vi "Read myTemp.vi"(6 "Reset Time":bool, 8 "error in (no error)":errorcluster, 9 "myTemp Setup":T1={"Offset Temp"=0.0, "Set Offset"=FALSE, "Calibration Data"=[{"Ka"=0.000739984, "Kb"=0.000278736, "Kc"=9.26322e-08}, {"Ka"=0.00073998, "Kb"=0.00027874, "Kc"=9.2632e-08}, {"Ka"=0.00073998, "Kb"=0.00027874, "Kc"=9.2632e-08}, {"Ka"=0.00073998, "Kb"=0.00027874, "Kc"=9.2632e-08}, {"Ka"=0.00073998, "Kb"=0.00027874, "Kc"=9.2632e-08}, {"Ka"=0.00073998, "Kb"=0.00027874, "Kc"=9.2632e-08}, {"Ka"=0.00073998, "Kb"=0.00027874, "Kc"=9.2632e-08}], "Chan Select"=[TRUE, TRUE, TRUE, FALSE, FALSE, FALSE, FALSE], "Clear Offsets"=FALSE, "Input Mode"=FALSE, "Chart History Length"=2000, "Use One K Set"=TRUE} {"Chart History Length" min=1 max=10000 step=1; "Calibration Data"."Kc" format="%#.4e"; "Calibration Data"."Kb" format="%#.4e"; "Calibration Data"."Ka" format="%#.4e"; "Offset Temp" min=-40.0 max=250.0 step=1.0}, 11 "task array in":refnum<k21>[](array[refnum])) -> (0 "error out":errorcluster, 1 "Elapsed Time":dbl, 2 "temperature values (°C)":dbl[](array[numeric]), 3 "task array out":refnum<k21>[](array[refnum]), 5 "XY Graph":cluster{"X":dbl[], "Y":dbl[]}[](array[cluster]))   [LabVIEW 2013]
doc: "This subVI is designed to control the multiplexor on the PITSCO myTemp so it can read in up to 7 temperature values. It use Steinhart non-linear scaling to convert the voltage measurements to temperature in °C."
uses:
  <vilib>/DAQmx/write.llb/DAQmx Write (Digital 1D Bool NChan 1Samp 1Line).vi
  <vilib>/DAQmx/read.llb/DAQmx Read (Analog 1D Wfm NChan NSamp).vi
  <vilib>/Analysis/baseanly.llb/Mean (DBL).vi
  <vilib>/DAQmx/miscellaneous.llb/DAQmx Fill In Error Info.vi
  <vilib>/Analysis/NI_AALBase.lvlib
panel:
  # "Select Temperature Channels to Display"
  # "Temp1"
  # "Temp2"
  # "Temp3"
  # "Temp4"
  # "Temp5"
  # "Temp6"
  # "Temp7"
  # "Null Temperature Setting"
  # "Calibration Coefficients"
  # "Temp1"
  # "Temp2"
  # "Temp3"
  # "Temp4"
  # "Temp5"
  # "Temp6"
  # "Temp7"
  # "Ka"
  # "Kb"
  # "Kc"
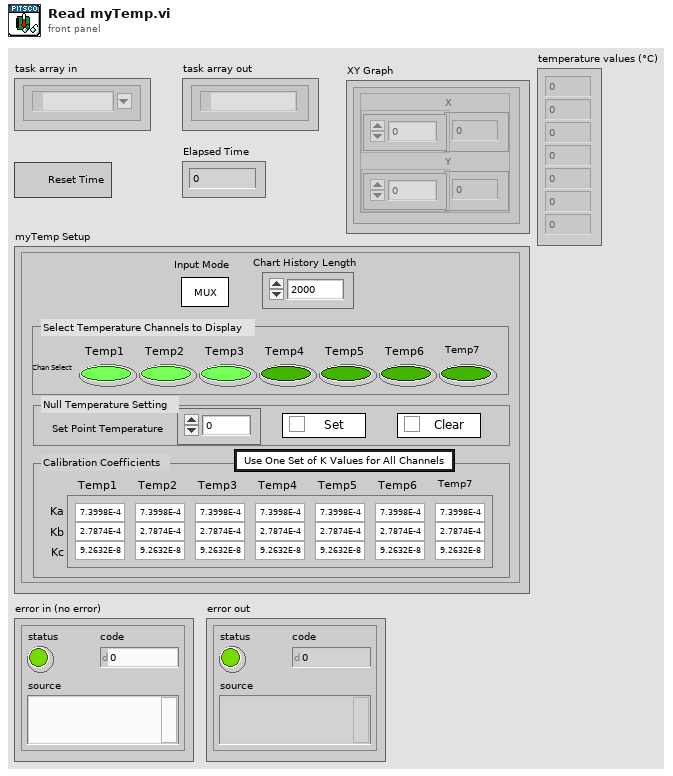
[diagram p1: front panel]
types:
  T1 = cluster{"Offset Temp":dbl, "Set Offset":bool, "Calibration Data":cluster{"Ka":dbl, "Kb":dbl, "Kc":dbl}[], "Chan Select":bool[], "Clear Offsets":bool, "Input Mode":bool, "Chart History Length":i32, "Use One K Set":bool}
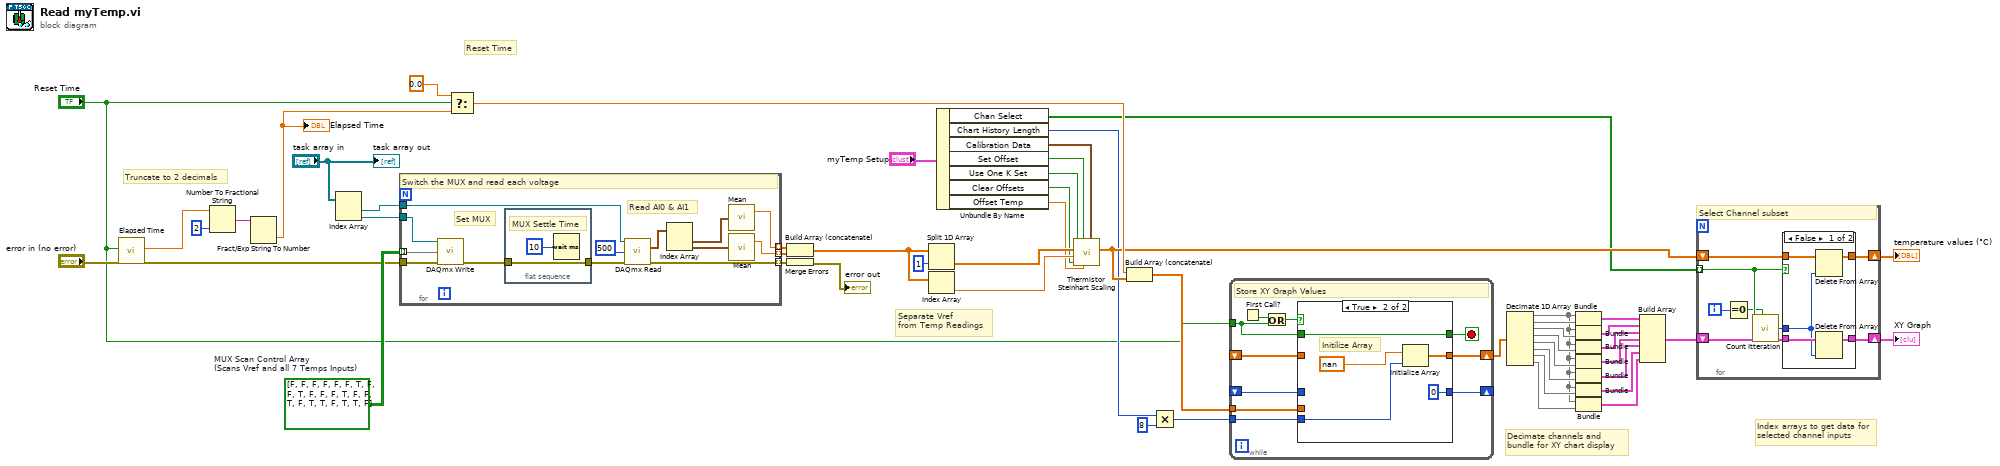
[diagram p0: block diagram]
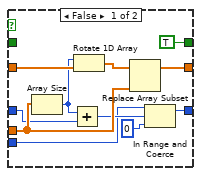
[diagram p2: hidden frame]
diagram:
  w37 = bool[][] [[FALSE, FALSE, FALSE, FALSE, FALSE, FALSE], [TRUE, FALSE, FALSE, TRUE, FALSE, FALSE], [FALSE, TRUE, FALSE, FALSE, TRUE, FALSE], [TRUE, TRUE, FALSE, TRUE, TRUE, FALSE]]  # MUX Scan Control Array (Scans Vref and all 7 Temps Inputs)
  # "Reset Time"
  # "Truncate to 2 decimals"
  # "Separate Vref\nfrom Temp Readings"
  # "Index arrays to get data for\nselected channel inputs"
  # "Decimate channels and \nbundle for XY chart display"
  n1 = call "Elapsed Time"("Reset"="Reset Time", "error in (no error)"="error in (no error)") -> ("Elapsed Time (s)"=w14:dbl, "error out"=w15:errorcluster)  [unwired: 10 in, 6 out]
  n2 = Number To Fractional String(number=w14, precision (6)=i16 2 ("precision (3)")) -> (F-format string=w17:string)  [unwired: 2 in]
  n3 = Fract/Exp String To Number(string=w17) -> (number=w8:dbl)  [unwired: 3 in, 1 out]
  "Elapsed Time" <- w8
  n4 = Index Array(array="task array in") -> (element #1=w6:refnum<k21>, element #2=w7:refnum<k21>)  [unwired: 2 in]
  n5 = for {
    tunnel: [w59] -> w39 mode=indexing
    tunnel: w37 -> [w58] mode=indexing
    tunnel: [w54] -> w41 mode=indexing
    tunnel: [w53] -> w40 mode=indexing
    tunnel: w15 -> [w61]
    tunnel: w7 -> [w65]
    tunnel: w6 -> [w63]
    # "Read AI0 & AI1"
    # "Set MUX"
    # "Switch the MUX and read each voltage"
    n6 = call-poly <vilib>:"DAQmx Write.vi"("task/channels in"=w65, "data"=w58, "error in"=w61) -> ("error out"=w60:errorcluster)  [unwired: 10 in, 2 out]
    n7 = flat-sequence {
      tunnel: w60 -> [w67]
      tunnel: [w67] -> w62
      frame #0 {
        # "MUX Settle Time"
        n8 = Wait (ms)(milliseconds to wait=u32 10) -> ()  [unwired: 1 out]
      }
    }
    n9 = call-poly <vilib>:"DAQmx Read.vi"("task/channels in"=w63, "number of samples per channel"=500, "error in"=w62) -> ("data"=w57:waveform(dbl)[], "error out"=w59:errorcluster)  [unwired: 10 in, 1 out]
    n10 = Index Array(array=w57) -> (element #1=w56:waveform(dbl), element #2=w55:waveform(dbl))  [unwired: 2 in]
    n11 = call-poly <vilib>:"Mean.vi"("X"=w56) -> ("mean"=w54:dbl)  [unwired: 1 out]
    n12 = call-poly <vilib>:"Mean.vi"("X"=w55) -> ("mean"=w53:dbl)  [unwired: 1 out]
  }
  n13 = Select(t=0.0, s="Reset Time", f=w8) -> (s? t:f=w51:dbl)
  n14 = Build Array (concatenate)(w41, w40) -> (w44:dbl[])
  n15 = Merge Errors(w39) -> (→"error out":errorcluster)
  n16 = Split 1D Array(array=w44, index=1) -> (second subarray=w42:dbl[])  [unwired: 1 out]
  n17 = Index Array(array=w44) -> (element=w46:dbl)  [unwired: 1 in]
  n18 = Unbundle By Name("myTemp Setup") -> ("Chan Select"=w20:bool[], "Chart History Length"=w21:i32, "Calibration Data"=w47:cluster{"Ka":dbl, "Kb":dbl, "Kc":dbl}[], "Set Offset"=w48:bool, "Use One K Set"=w43:bool, "Clear Offsets"=w18:bool, "Offset Temp"=w19:dbl)
  n19 = call "Thermistor Steinhart Scaling.vi"("Calibration Coefficients"=w47, "Set Point Temp"=w19, "Set"=w48, "Clear"=w18, "Vref"=w46, "Vt Measured"=w42, "Use One K Set"=w43) -> ("Temps"=w38:dbl[])  [unwired: 3 in, 1 out]
  n20 = Build Array (concatenate)(w51, w38) -> (w4:dbl[])
  n21 = Multiply(x=w21, y=8) -> (x*y=w2:i32)
  n22 = while {
    tunnel: w2 -> [w77]
    shift-right: [w76] -> w1
    shift-left: _ -> [w75]
    tunnel: w4 -> [w74]
    shift-right: [w70] -> _
    shift-left: _ -> [w69]
    tunnel: "Reset Time" -> [w68]
    stop <- w71 stop-if-true
    # "Store XY Graph Values"
    n23 = First Call?() -> (First Call?: T/F=w73:bool)
    n24 = Or(x=w73, y=w68) -> (x .or. y?=w72:bool)
    n25 = case shown="True" w72 {
      tunnel: w77 -> [w80 w93]
      tunnel: [w86 w91] -> w76
      tunnel: w75 -> [w88 _]
      tunnel: w74 -> [w85 _]
      tunnel: [TRUE w90] -> w71
      tunnel: w68 -> [_ w90]
      tunnel: [w78 0] -> w70
      tunnel: w69 -> [w83 _]
      frame False {
        n26 = Array Size(array=w85) -> (size(s)=w82:i32)
        n27 = Add(x=w82, y=w83) -> (x+y=w81:i32)
        n28 = Rotate 1D Array(1:w88, 2:w82) -> (0:w87:dbl[])
        n29 = Replace Array Subset(array=w87, new element=w85) -> (w86:dbl[])  [unwired: 1 in]
        n30 = In Range and Coerce(upper limit=w80, x=w81, lower limit=0) -> (coerced(x)=w78:i32)  [unwired: 1 out]
      }
      frame True {
        # "Initilize Array"
        n31 = Initialize Array(nan ("element"), w93) -> (w91:dbl[])
      }
    }
  }
  n32 = Decimate 1D Array(w1) -> (w22:dbl[], w23:dbl[], w24:dbl[], w25:dbl[], w26:dbl[], w27:dbl[], w28:dbl[], w29:dbl[])
  n33 = Bundle(w22, w23) -> (w30:cluster{dbl[], dbl[]})  [unwired: 1 in]
  n34 = Bundle(w22, w24) -> (w31:cluster{dbl[], dbl[]})  [unwired: 1 in]
  n35 = Bundle(w22, w25) -> (w32:cluster{dbl[], dbl[]})  [unwired: 1 in]
  n36 = Bundle(w22, w26) -> (w33:cluster{dbl[], dbl[]})  [unwired: 1 in]
  n37 = Bundle(w22, w27) -> (w34:cluster{dbl[], dbl[]})  [unwired: 1 in]
  n38 = Bundle(w22, w28) -> (w35:cluster{dbl[], dbl[]})  [unwired: 1 in]
  n39 = Bundle(w22, w29) -> (w36:cluster{dbl[], dbl[]})  [unwired: 1 in]
  n40 = Build Array(w30, w31, w32, w33, w34, w35, w36) -> (w49:cluster{dbl[], dbl[]}[])
  n41 = for {
    tunnel: w20 -> [w99] mode=indexing
    shift-right: [w100] -> w10
    shift-left: w49 -> [w101]
    shift-right: [w95] -> w11
    shift-left: w38 -> [w94]
    i -> [w97]
    # "Select Channel subset"
    n42 = Equal To 0?(x=w97) -> (x = 0?=w96:bool)
    n43 = call "Count Itteration.vi"("Reset"=w96, "Enable"=w99) -> ("Itteration"=w98:i32)  [unwired: 5 in, 1 out]
    n44 = case shown="False" w99 {
      tunnel: w101 -> [w106 w108]
      tunnel: [w105 w108] -> w100
      tunnel: w98 -> [w102 _]
      tunnel: [w104 w107] -> w95
      tunnel: w94 -> [w103 w107]
      frame False {
        n45 = Delete From Array(array=w103, index=w102) -> (array with subset deleted=w104:dbl[])  [unwired: 1 in, 1 out]
        n46 = Delete From Array(array=w106, index=w102) -> (array with subset deleted=w105:cluster{dbl[], dbl[]}[])  [unwired: 1 in, 1 out]
      }
      frame True {
      }
    }
  }
  "temperature values (°C)" <- w11
  "XY Graph" <- w10
  "task array out" <- "task array in"
